vi "计算流水号.vi"(0 "功能":enum16{"流水号归零", "计算流水号"}(ring), 5 "工位":string, 7 "产品名":string, 11 "error in":errorcluster) -> (4 "当前流水号":string, 15 "error out":errorcluster)   [LabVIEW 2016]
uses:
  <vilib>/Utility/config.llb/Write Key (String).vi
  <vilib>/Utility/config.llb/Read Key (String).vi
  <vilib>/Utility/config.llb/NI_LVConfig.lvlib
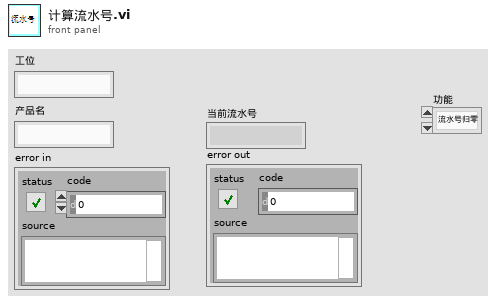
[diagram p1: front panel]
types:
  T1 = typedef "NI_LVConfig.lvlib/Config Data RefNum.ctl" = refnum<k1>
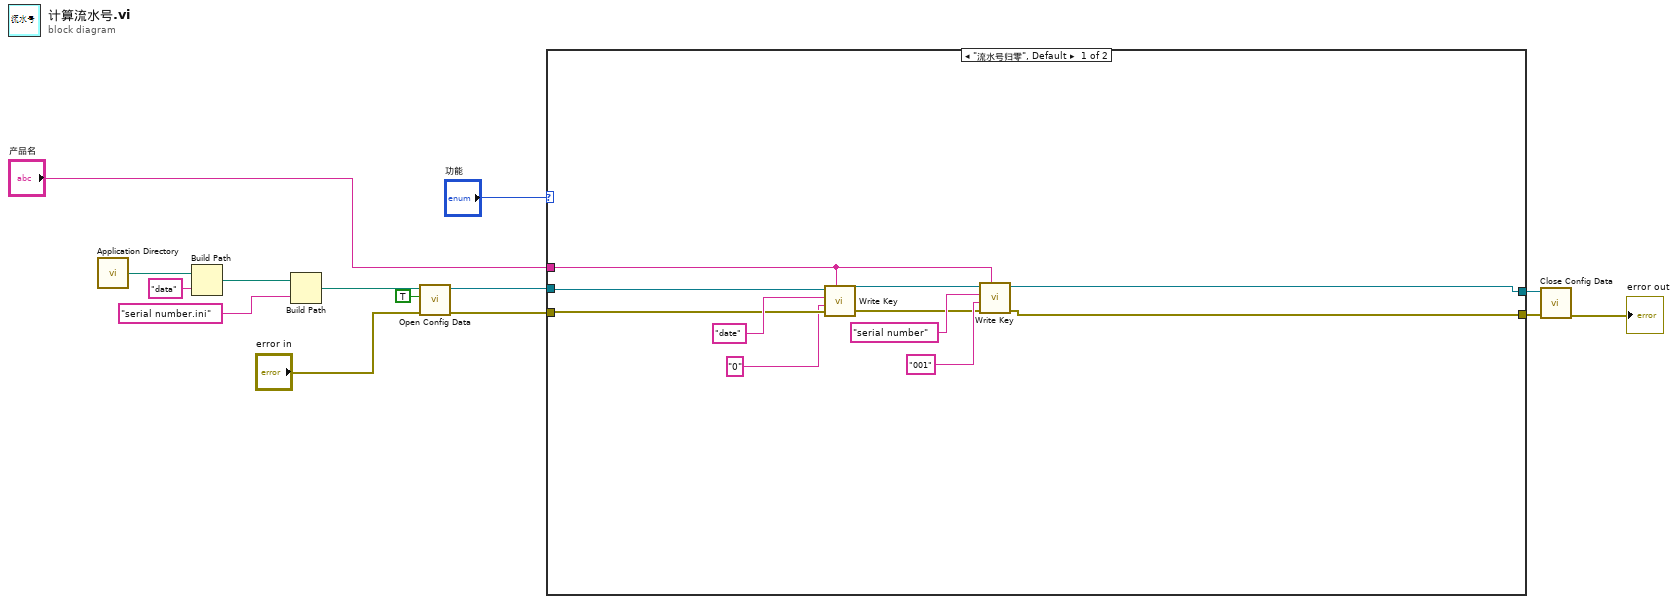
[diagram p0: block diagram]
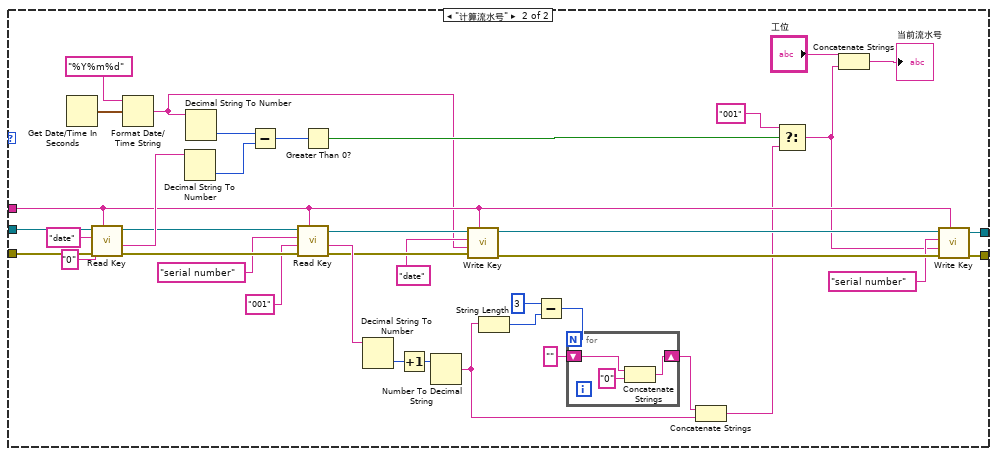
[diagram p2: hidden frame]
diagram:
  n1 = call <vilib>:"Application Directory.vi"() -> ("Application Directory"=w14:path)
  n2 = Build Path(base path=w14, name or relative path="data") -> (appended path=w12:path)
  n3 = Build Path(base path=w12, name or relative path="serial number.ini") -> (appended path=w10:path)
  n4 = call <vilib>:"Open Config Data.vi"("error in (no error)"="error in", "create file if necessary (T)"=TRUE, "configuration file path"=w10) -> ("error out"=w6:errorcluster, "refnum"=w7:T1)  [unwired: 6 in, 1 out]
  n5 = case shown="\"流水号归零\", Default" "功能" {
    tunnel: w7 -> [w24 w56]
    tunnel: w6 -> [w23 w55]
    tunnel: "产品名" -> [w20 w39]
    tunnel: [w15 w32] -> w4
    tunnel: [w16 w31] -> w3
    frame "流水号归零", Default {
      n6 = call-poly <vilib>:"Write Key.vi"("section"=w20, "error in (no error)"=w23, "value"="0" ("key"), "key"="date", "refnum"=w24) -> ("error out"=w17:errorcluster, "refnum out"=w21:T1)  [unwired: 4 in, 1 out]
      n7 = call-poly <vilib>:"Write Key.vi"("section"=w20, "error in (no error)"=w17, "value"="001" ("key"), "key"="serial number", "refnum"=w21) -> ("error out"=w16:errorcluster, "refnum out"=w15:T1)  [unwired: 4 in, 1 out]
    }
    frame "计算流水号" {
      n8 = Get Date/Time In Seconds() -> (seconds since 1Jan1904=w52:timestamp)
      n9 = call-poly <vilib>:"Read Key.vi"("section"=w39, "error in (no error)"=w55, "default value"="0", "key"="date", "refnum"=w56) -> ("error out"=w46:errorcluster, "value"=w50:string, "refnum out"=w47:T1)  [unwired: 3 in, 1 out]
      n10 = Format Date/Time String(time format string (%c)="%Y%m%d", seconds (now)=w52) -> (date/time string=w37:string)  [unwired: 1 in]
      n11 = Decimal String To Number(string=w50) -> (number=w48:i32)  [unwired: 2 in, 1 out]
      n12 = Decimal String To Number(string=w37) -> (number=w49:i32)  [unwired: 2 in, 1 out]
      n13 = Subtract(x=w49, y=w48) -> (x-y=w44:i32)
      n14 = call-poly <vilib>:"Read Key.vi"("section"=w39, "error in (no error)"=w46, "default value"="001", "key"="serial number", "refnum"=w47) -> ("error out"=w40:errorcluster, "value"=w42:string, "refnum out"=w41:T1)  [unwired: 3 in, 1 out]
      n15 = Greater Than 0?(x=w44) -> (x > 0?=w43:bool)
      n16 = Decimal String To Number(string=w42) -> (number=w64:i32)  [unwired: 2 in, 1 out]
      n17 = Increment(x=w64) -> (x+1=w63:i32)
      n18 = Number To Decimal String(number=w63) -> (decimal integer string=w58:string)  [unwired: 1 in]
      n19 = call-poly <vilib>:"Write Key.vi"("section"=w39, "error in (no error)"=w40, "value"=w37, "key"="date", "refnum"=w41) -> ("error out"=w34:errorcluster, "refnum out"=w35:T1)  [unwired: 4 in, 1 out]
      n20 = String Length(string=w58) -> (length=w62:i32)
      n21 = Subtract(x=3, y=w62) -> (x-y=w60:i32)
      n22 = for {
        N: w60 -> [_]
        shift-right: [w66] -> w59
        shift-left: "" -> [w67]
        n23 = Concatenate Strings(w67, "0" ("string")) -> (w66:string)
      }
      n24 = Concatenate Strings(w59, w58) -> (w28:string)
      n25 = Select(t="001" ("f"), s=w43, f=w28) -> (s? t:f=w27:string)
      n26 = Concatenate Strings("工位", w27) -> (→"当前流水号":string)
      n27 = call-poly <vilib>:"Write Key.vi"("section"=w39, "error in (no error)"=w34, "value"=w27, "key"="serial number", "refnum"=w35) -> ("error out"=w31:errorcluster, "refnum out"=w32:T1)  [unwired: 4 in, 1 out]
    }
  }
  n28 = call <vilib>:"Close Config Data.vi"("error in (no error)"=w3, "refnum"=w4) -> ("error out"=→"error out":errorcluster)  [unwired: 8 in, 1 out]
